vi "Sortrecipestypes.vi"(8 "error in (no error)":errorcluster, 10 "RecipeFolderPath":path, 11 "TopLevel.lvclass":refnum<class "TopLevel.lvclass">) -> (0 "error out":errorcluster, 1 "Products":string[](array[string]), 2 "Design Print Recipes":path[](array[path]), 3 "reference out":refnum<class "TopLevel.lvclass">, 4 "DebugDict":T1)   [LabVIEW 2022 SP3]
uses:
  Classes/TopLevel/TopLevel.lvclass
  <vilib>/TELLC/Dynamic CVT API/TD Dynamic CVT DVR--ref.ctl
  Controls/RecipesFolderSummary--Cluster.ctl
  Controls/DLP RecipeTypesData--Cluster.ctl
  Controls/RecipeInfo--Cluster.ctl
  <vilib>/xml/Load XML File.vi
  <vilib>/xml/Close Reference(Node).vi
  <userlib>/_OpenG.lib/array/array.llb/Remove Duplicates from 1D Array (String)__ogtk.vi
  <userlib>/_OpenG.lib/array/array.llb/Search 1D Array (String)__ogtk.vi
  <userlib>/_OpenG.lib/array/array.llb/Index 1D Array Elements (String)__ogtk.vi
  <userlib>/_OpenG.lib/array/array.llb/Index 1D Array Elements (Path)__ogtk.vi
  <userlib>/_OpenG.lib/array/array.llb/Remove Duplicates from 1D Array (Path)__ogtk.vi
  <vilib>/xml/NI_XML.lvlib
  <resource>/objmgr/DOMUserDefRef.rc
panel:
  out "PrintDesignProducts":string[](array[string])
  out "CalibrationProducts":string[](array[string])
  out "RecipeNames":string[](array[string])
  out "Calibration Recipes":path[](array[path])
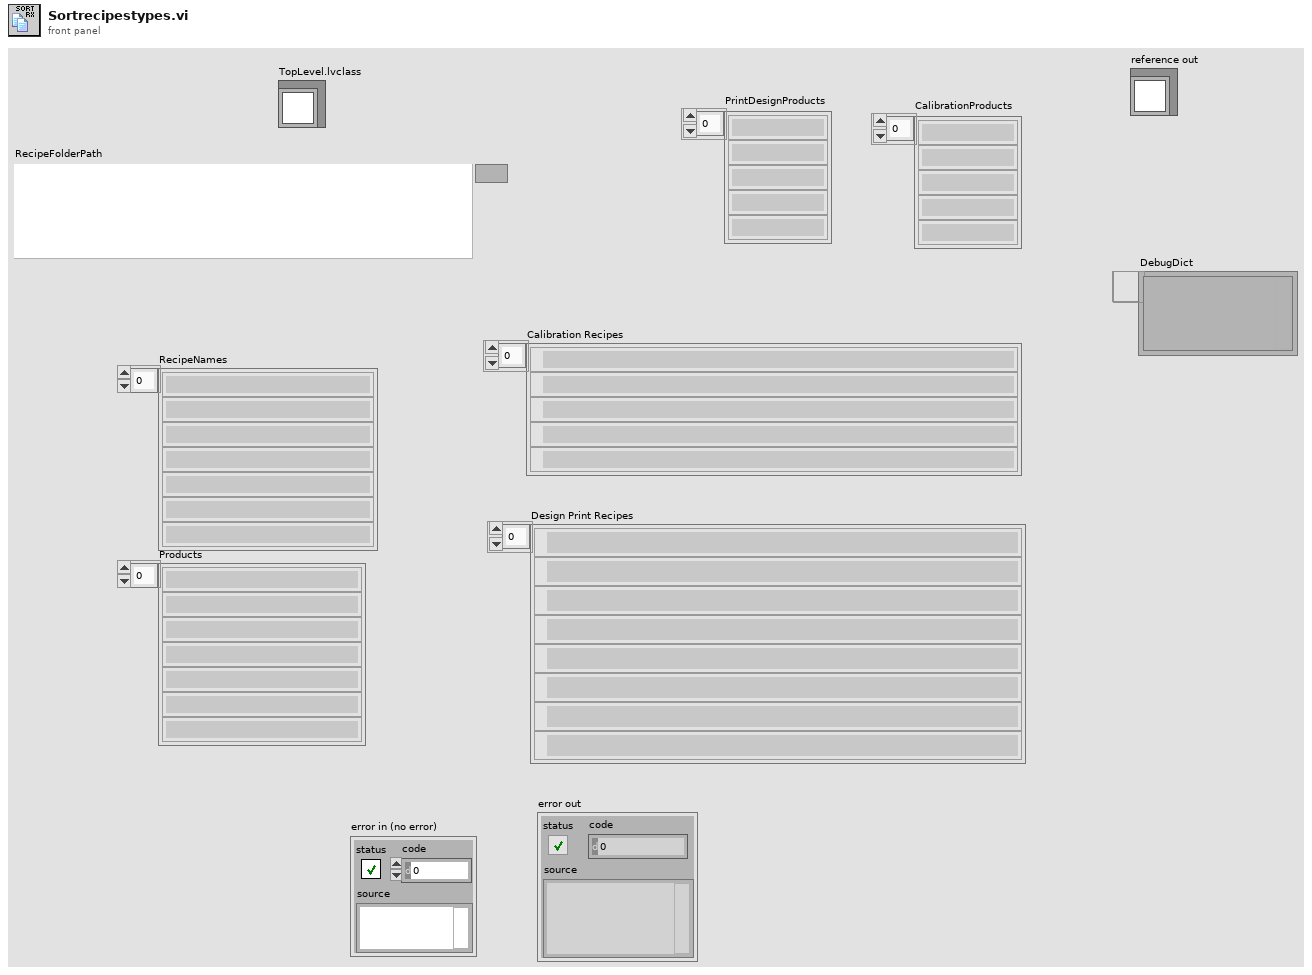
[diagram p1: front panel]
types:
  T1 = typedef "TD Dynamic CVT DVR--ref.ctl" = refnum<data-value>
  T2 = typedef "RecipesFolderSummary--Cluster.ctl" = cluster{"Products":string[], "RecipeTypes":string[]}
  T3 = typedef "DLP RecipeTypesData--Cluster.ctl" = cluster{"Product":string, "RecipePathsByProduct":path[], "RecipeNamesByProduct":string[]}
  T4 = typedef "RecipeInfo--Cluster.ctl" = cluster{"Path":path, "Type":string, "Product":string}
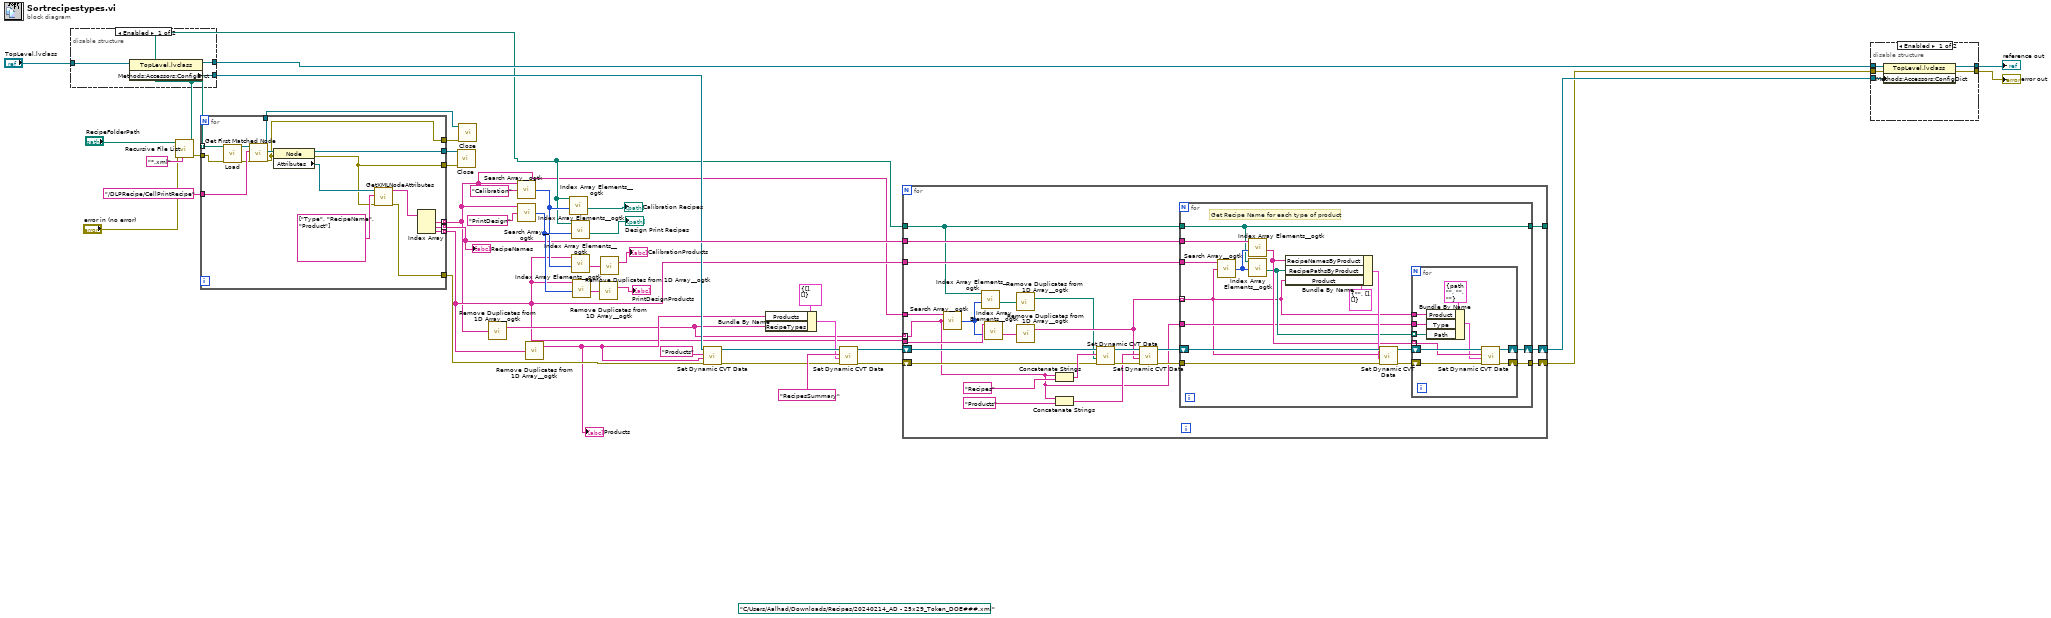
[diagram p0: block diagram]
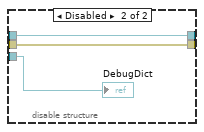
[diagram p2: hidden frame]
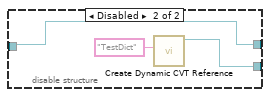
[diagram p3: hidden frame]
diagram:
  (unwired) path "C:/Users/Aalhad/Downloads/Recipes/20240214_AD - 25x29_Token_DOE###.xml"
  n1 = disable-structure shown="Enabled" {
    disable-tunnel: [w44 w47] -> w18
    disable-tunnel: [w43 w45] -> w17
    disable-tunnel: "TopLevel.lvclass" -> [w42 w45]
    frame Enabled {
      n2 = property class="TopLevel.lvclass"(reference=w42) -> (reference out=w43:refnum<class "TopLevel.lvclass">, "Methods:Accessors:ConfigDict"=w44:T1)  [unwired: 1 in, 1 out]
    }
    frame Disabled {
      n3 = call <vilib>:"Create Dynamic CVT Reference.vi"("DictName"="TestDict") -> ("dCVT DVR out"=w47:T1)  [unwired: 9 in, 1 out]
    }
  }
  n4 = call <vilib>:"Recursive File List.vi"("pattern"="*.xml", "error in (no error)"="error in (no error)", "Folder Path"="RecipeFolderPath") -> ("error out"=w35:errorcluster, "All Files in Dir"=w5:path[])  [unwired: 4 in, 3 out]
  n5 = for {
    tunnel: w5 -> [w64] mode=indexing
    tunnel: "/DLPRecipe/CellPrintRecipe" ("XPath Expression") -> [w62]
    tunnel: [w54] -> w1 mode=indexing
    tunnel: w35 -> [w58]
    tunnel: [w56] -> w14
    tunnel: [w53] -> w25 mode=indexing
    tunnel: [w52] -> w2 mode=indexing
    tunnel: [w51] -> w30
    tunnel: [w50] -> w29
    tunnel: [w49] -> w28
    tunnel: [w48] -> w27
    n6 = call-poly <vilib>:"Load.vi"("path to XML document"=w64, "error in (no error)"=w58) -> ("DOM document out"=w63:refnum<k20>, "error out"=w57:errorcluster)  [unwired: 11 in, 1 out]
    n7 = call <vilib>:"Get First Matched Node.vi"("error in (no error)"=w57, "XPath expression"=w62, "node in"=w63) -> ("error out"=w51:errorcluster, "node result"=w61:refnum<k20>, "node out"=w50:refnum<k20>)  [unwired: 6 in]
    n8 = property class="Node"(reference=w61, error in=w51) -> (reference out=w48:refnum<k20>, error out=w49:errorcluster, "Attributes"=w60:refnum<k20>)
    n9 = call "GetXMLNodeAttributes.vi"("error in (no error)"=w49, "ArributeNames"=string[] ["Type", "RecipeName", "Product"], "AtrributesRefIn"=w60) -> ("error out"=w56:errorcluster, "AttributeValues"=w59:string[])  [unwired: 7 in]
    n10 = Index Array(array=w59) -> (element #1=w54:string, element #2=w53:string, element #3=w52:string)  [unwired: 3 in]
  }
  "RecipeNames" <- w25
  n11 = call-poly <vilib>:"Close.vi"("error in (no error)"=w28, "node"=w27) -> ()  [unwired: 8 out]
  n12 = call-poly <vilib>:"Close.vi"("error in (no error)"=w30, "node"=w29) -> ()  [unwired: 8 out]
  n13 = call-poly <userlib>:"Remove Duplicates from 1D Array__ogtk.vi"("Input Array"=w1) -> ("Output Array"=w3:string[])  [unwired: 1 out]
  n14 = call-poly <userlib>:"Search Array__ogtk.vi"("Array"=w1, "Element Data"="Calibration" ("slice")) -> ("Indices of Elements"=w31:i32[])  [unwired: 7 in]
  n15 = call-poly <userlib>:"Search Array__ogtk.vi"("Array"=w1, "Element Data"="PrintDesign" ("slice")) -> ("Indices of Elements"=w32:i32[])  [unwired: 7 in]
  n16 = call-poly <userlib>:"Remove Duplicates from 1D Array__ogtk.vi"("Input Array"=w2) -> ("Output Array"=w10:string[])  [unwired: 1 out]
  "Products" <- w10
  n17 = call-poly <userlib>:"Index Array Elements__ogtk.vi"("indices"=w31, "array"=w5) -> ("elements"=→"Calibration Recipes":path[])  [unwired: 9 in]
  n18 = call-poly <userlib>:"Index Array Elements__ogtk.vi"("indices"=w32, "array"=w5) -> ("elements"=→"Design Print Recipes":path[])  [unwired: 9 in]
  n19 = call-poly <userlib>:"Index Array Elements__ogtk.vi"("indices"=w31, "array"=w2) -> ("elements"=w34:string[])  [unwired: 9 in]
  n20 = call-poly <userlib>:"Index Array Elements__ogtk.vi"("indices"=w32, "array"=w2) -> ("elements"=w33:string[])  [unwired: 9 in]
  n21 = call-poly <userlib>:"Remove Duplicates from 1D Array__ogtk.vi"("Input Array"=w33) -> ("Output Array"=→"PrintDesignProducts":string[])  [unwired: 1 out]
  n22 = call-poly <userlib>:"Remove Duplicates from 1D Array__ogtk.vi"("Input Array"=w34) -> ("Output Array"=→"CalibrationProducts":string[])  [unwired: 1 out]
  n23 = call <vilib>:"Set Dynamic CVT Data.vi"("error in (no error)"=w14, "value"=w10, "DataName"="Products", "dCVT DVR"=w18) -> ("error out"=w13:errorcluster, "dCVT DVR out"=w22:T1)  [unwired: 5 in, 1 out]
  n24 = Bundle By Name(cluster=T2 {"Products"=[], "RecipeTypes"=[]}, "Products"=w10, "RecipeTypes"=w3) -> (w11:T2)
  n25 = call <vilib>:"Set Dynamic CVT Data.vi"("error in (no error)"=w13, "value"=w11, "DataName"="RecipesSummary" ("String"), "dCVT DVR"=w22) -> ("error out"=w20:errorcluster, "dCVT DVR out"=w21:T1)  [unwired: 5 in, 1 out]
  n26 = for {
    tunnel: w25 -> [w87]
    tunnel: w2 -> [w85]
    tunnel: w5 -> [w82]
    tunnel: [w84] -> _
    shift-right: [w88] -> w26
    shift-left: w21 -> [w79]
    shift-right: [w86] -> w24
    shift-left: w20 -> [w72]
    tunnel: w3 -> [w65] mode=indexing
    tunnel: w1 -> [w83]
    tunnel: w2 -> [w81]
    n27 = call-poly <userlib>:"Search Array__ogtk.vi"("Array"=w83, "Element Data"=w65) -> ("Indices of Elements"=w80:i32[])  [unwired: 7 in]
    n28 = call-poly <userlib>:"Index Array Elements__ogtk.vi"("indices"=w80, "array"=w82) -> ("elements"=w67:path[])  [unwired: 9 in]
    n29 = call-poly <userlib>:"Index Array Elements__ogtk.vi"("indices"=w80, "array"=w81) -> ("elements"=w69:string[])  [unwired: 9 in]
    n30 = call-poly <userlib>:"Remove Duplicates from 1D Array__ogtk.vi"("Input Array"=w67) -> ("Output Array"=w66:path[])  [unwired: 1 out]
    n31 = call-poly <userlib>:"Remove Duplicates from 1D Array__ogtk.vi"("Input Array"=w69) -> ("Output Array"=w68:string[])  [unwired: 1 out]
    n32 = Concatenate Strings(w65, "Recipes" ("string")) -> (w76:string)
    n33 = Concatenate Strings(w65, "Products" ("string")) -> (w70:string)
    n34 = call <vilib>:"Set Dynamic CVT Data.vi"("error in (no error)"=w72, "value"=w66, "DataName"=w76, "dCVT DVR"=w79) -> ("error out"=w73:errorcluster, "dCVT DVR out"=w75:T1)  [unwired: 5 in, 1 out]
    n35 = call <vilib>:"Set Dynamic CVT Data.vi"("error in (no error)"=w73, "value"=w68, "DataName"=w70, "dCVT DVR"=w75) -> ("error out"=w71:errorcluster, "dCVT DVR out"=w74:T1)  [unwired: 5 in, 1 out]
    n36 = for {
      tunnel: w68 -> [w89] mode=indexing
      tunnel: w85 -> [w104]
      tunnel: w82 -> [w97]
      tunnel: w87 -> [w103]
      shift-right: [w95] -> w88
      shift-left: w74 -> [w100]
      tunnel: [w93] -> w86
      tunnel: w71 -> [w98]
      tunnel: [w97] -> w84
      tunnel: w65 -> [w90]
      # "Get Recipe Name for each type of product"
      n37 = call-poly <userlib>:"Search Array__ogtk.vi"("Array"=w104, "Element Data"=w89) -> ("Indices of Elements"=w102:i32[])  [unwired: 7 in]
      n38 = call-poly <userlib>:"Index Array Elements__ogtk.vi"("indices"=w102, "array"=w103) -> ("elements"=w92:string[])  [unwired: 9 in]
      n39 = call-poly <userlib>:"Index Array Elements__ogtk.vi"("indices"=w102, "array"=w97) -> ("elements"=w91:path[])  [unwired: 9 in]
      n40 = Bundle By Name(cluster=T3 {"Product"="", "RecipePathsByProduct"=[], "RecipeNamesByProduct"=[]}, "RecipeNamesByProduct"=w92, "RecipePathsByProduct"=w91, "Product"=w89) -> (w99:T3)
      n41 = call <vilib>:"Set Dynamic CVT Data.vi"("error in (no error)"=w98, "value"=w99, "DataName"=w89, "dCVT DVR"=w100) -> ("error out"=w94:errorcluster, "dCVT DVR out"=w96:T1)  [unwired: 5 in, 1 out]
      n42 = for {
        shift-right: [w113] -> w95
        shift-left: w96 -> [w114]
        shift-right: [w111] -> w93
        shift-left: w94 -> [w112]
        tunnel: w92 -> [w110] mode=indexing
        tunnel: w91 -> [w106] mode=indexing
        tunnel: w90 -> [w109]
        tunnel: w89 -> [w107]
        n43 = Bundle By Name(cluster=T4 {"Path"=path "", "Type"="", "Product"=""} ("RecipeInfo"), "Product"=w107, "Type"=w109, "Path"=w106) -> (w108:T4)
        n44 = call <vilib>:"Set Dynamic CVT Data.vi"("error in (no error)"=w112, "value"=w108, "DataName"=w110, "dCVT DVR"=w114) -> ("error out"=w111:errorcluster, "dCVT DVR out"=w113:T1)  [unwired: 5 in, 1 out]
      }
    }
  }
  n45 = disable-structure shown="Enabled" {
    disable-tunnel: w17 -> [w119 w121]
    disable-tunnel: w26 -> [w118 w122]
    disable-tunnel: [w117 w121] -> w16
    disable-tunnel: w24 -> [w116 w120]
    disable-tunnel: [w115 w120] -> w12
    frame Enabled {
      n46 = property class="TopLevel.lvclass"(reference=w119, error in=w116, "Methods:Accessors:ConfigDict"=w118) -> (reference out=w117:refnum<class "TopLevel.lvclass">, error out=w115:errorcluster)
    }
    frame Disabled {
      "DebugDict" <- w122
    }
  }
  "error out" <- w12
  "reference out" <- w16
